vi "u64 to cpx str.vi"(11 "Numeric":u64) -> (3 "String":string)   [LabVIEW 2020]
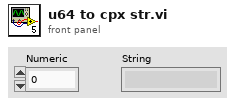
[diagram p1: front panel]
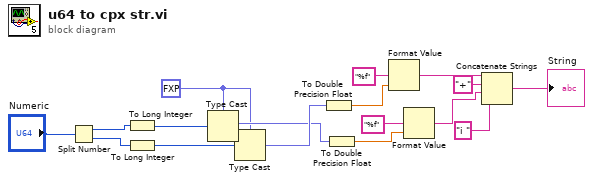
[diagram p0: block diagram]
diagram:
  w4 = fxp<+/-,32,11> 0.0 ("Number of Elements")
  n1 = Split Number(x="Numeric") -> (hi(x)=w1:u32, lo(x)=w2:u32)
  n2 = To Long Integer(number=w1) -> (32bit integer=w3:i32)
  n3 = To Long Integer(number=w2) -> (32bit integer=w15:i32)
  n4 = Type Cast(type=w4, x=w3) -> (*(type *) &x=w6:fxp<+/-,32,11>)
  n5 = Type Cast(type=w4, x=w15) -> (*(type *) &x=w16:fxp<+/-,32,11>)
  n6 = To Double Precision Float(number=w16) -> (double precision float=w7:dbl)
  n7 = To Double Precision Float(number=w6) -> (double precision float=w9:dbl)
  n8 = Format Value(format string="%f", value (0)=w7) -> (output string=w10:string)  [unwired: 1 in]
  n9 = Format Value(format string="%f", value (0)=w9) -> (output string=w12:string)  [unwired: 1 in]
  n10 = Concatenate Strings(w10, "+" ("string"), w12, "i " ("string")) -> (→"String":string)
